vi "Autonomous Independent.vi"   [LabVIEW 2013]
doc: "This VI is called when autonomous begins, and will automatically be terminated when autonomous ends. You can carry out timed or sensor driven robot movement independently without needing to return to the caller."
uses:
  <vilib>/Rock Robotics/WPI/Solenoid/WPI_SolenoidValue.ctl
  Robot Global Data.vi
  <vilib>/Rock Robotics/WPI/RobotDrive/WPI_RobotDriveGetSetRefNum.vi
  <vilib>/Rock Robotics/WPI/Solenoid/WPI_SolenoidSetEnum.vi
  <vilib>/Rock Robotics/WPI/RobotDrive/WPI_RobotDriveArcadeDrive_Standard(NoSaturation).vi
  <vilib>/Rock Robotics/WPI/Solenoid/Deprecated/WPI_SolenoidGetBool.vi
  <vilib>/Rock Robotics/WPI/Joystick/WPI_JoystickGetSetRefNum.vi
panel:
  # "Be sure to right-click and choose Data Operations>>Make Current Value default if you want to save the array values with the VI"
types:
  T1 = typedef "WPI_JoystickDevRef.ctl" = cluster{"Device":T2}
  T2 = typedef "WPI_JoystickDeviceEnum.ctl" = enum16{"USB 1", "USB 2", "USB 3", "USB 4", "Kinect 1", "Kinect 2"}
  T3 = cluster{"axis 1 (x)":dbl, "axis 2 (y)":dbl, "axis 3 (throttle)":dbl, "axis 4":dbl, "axis 5":dbl, "axis 6":dbl}
  T4 = typedef "WPI_SolenoidValue.ctl" = enum16{"Off", "On", "Forward", "Reverse"}
  T5 = typedef "WPI_MotorControlDeviceRef.ctl" = cluster{"DeviceStatus":errorcluster, "Type":enum16{"PWM", "CAN"}, "PWM":cluster{"Digital Module":T6, "PWM Channel":T7, "DeadBand":T8}, "CAN":cluster{"Device Number":u8, "Control Mode":T9, "Semaphore":T10, "Max Vout":dbl}, "Invert":bool, "TransformRef":T11, "InvTransformRef":T11}
  T6 = typedef "FPGA_TypedefDigitalModule.ctl" = enum16{"Digital Module 1", "Digital Module 2"}
  T7 = typedef "FPGA_DIOPWMChannel.ctl" = enum8{"PWM 1", "PWM 2", "PWM 3", "PWM 4", "PWM 5", "PWM 6", "PWM 7", "PWM 8", "PWM 9", "PWM 10", "Invalid"}
  T8 = typedef "WPI_PWMDeadband.ctl" = cluster{"Name":string, "maxPositivePwm":i32, "minPositivePwm":i32, "centerPwm":i32, "maxNegativePwm":i32, "minNegativePwm":i32, "angularRange":u16}
  T9 = typedef "WPI_CANJaguar_ControlMode.ctl" = enum8{"Percent VBus", "Current", "Speed", "Position", "Voltage"}
  T10 = typedef "Semaphore RefNum" = refnum<k1>
  T11 = typedef "WPI_PWMTransform_ConPane.ctl" = refnum<vi>
  T12 = typedef "WPI_SolenoidDevRef.ctl" = cluster{"DevStatus":errorcluster, "Solenoid Module":T13, "Forward Solenoid Channel":T14, "Reverse Solenoid Channel":T14}
  T13 = typedef "FPGA_TypedefSolenoidModule.ctl" = enum16{"Solenoid Module 1", "Solenoid Module 2"}
  T14 = typedef "WPI_SolenoidChannel.ctl" = enum8{"Solenoid 1", "Solenoid 2", "Solenoid 3", "Solenoid 4", "Solenoid 5", "Solenoid 6", "Solenoid 7", "Solenoid 8", "Invalid"}
  T15 = typedef "WPI_DigitalInputDevRef.ctl" = cluster{"DevStatus":errorcluster, "DIO Channel":T16, "Digital Module":T6}
  T16 = typedef "FPGA_DIOChannel.ctl" = enum8{"DIO 1", "DIO 2", "DIO 3", "DIO 4", "DIO 5", "DIO 6", "DIO 7", "DIO 8", "DIO 9", "DIO 10", "DIO 11", "DIO 12", "DIO 13", "DIO 14", "Invalid"}
  T17 = typedef "WPI_RobotDriveDevRef.ctl" = cluster{"DevStatus":errorcluster, "Motors[]":T5[], "Square Inputs":bool, "Max Output":dbl, "Isochronous":bool}
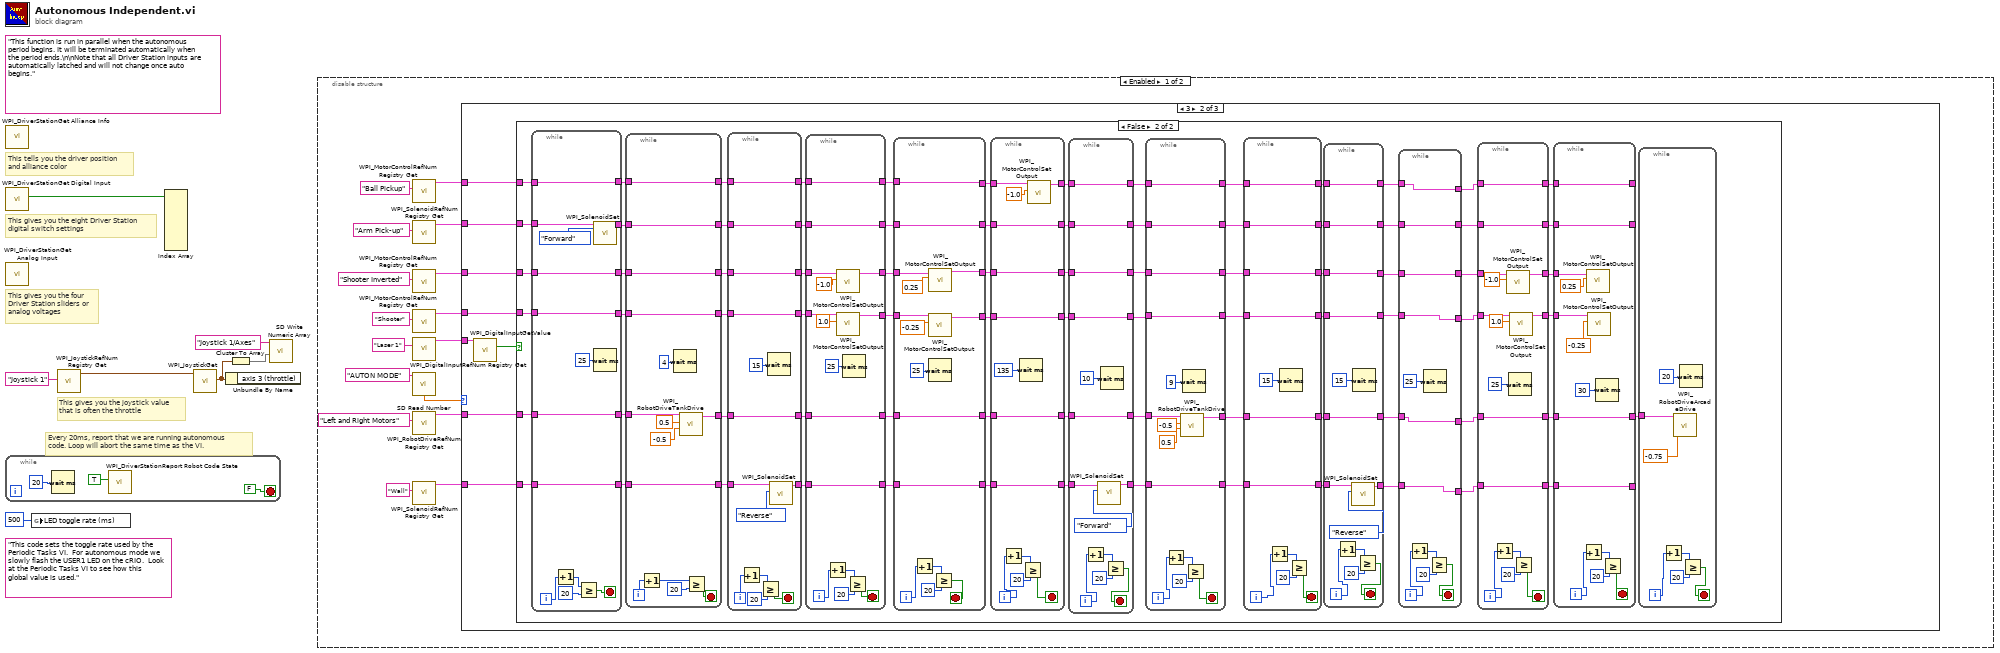
[diagram p0: block diagram]
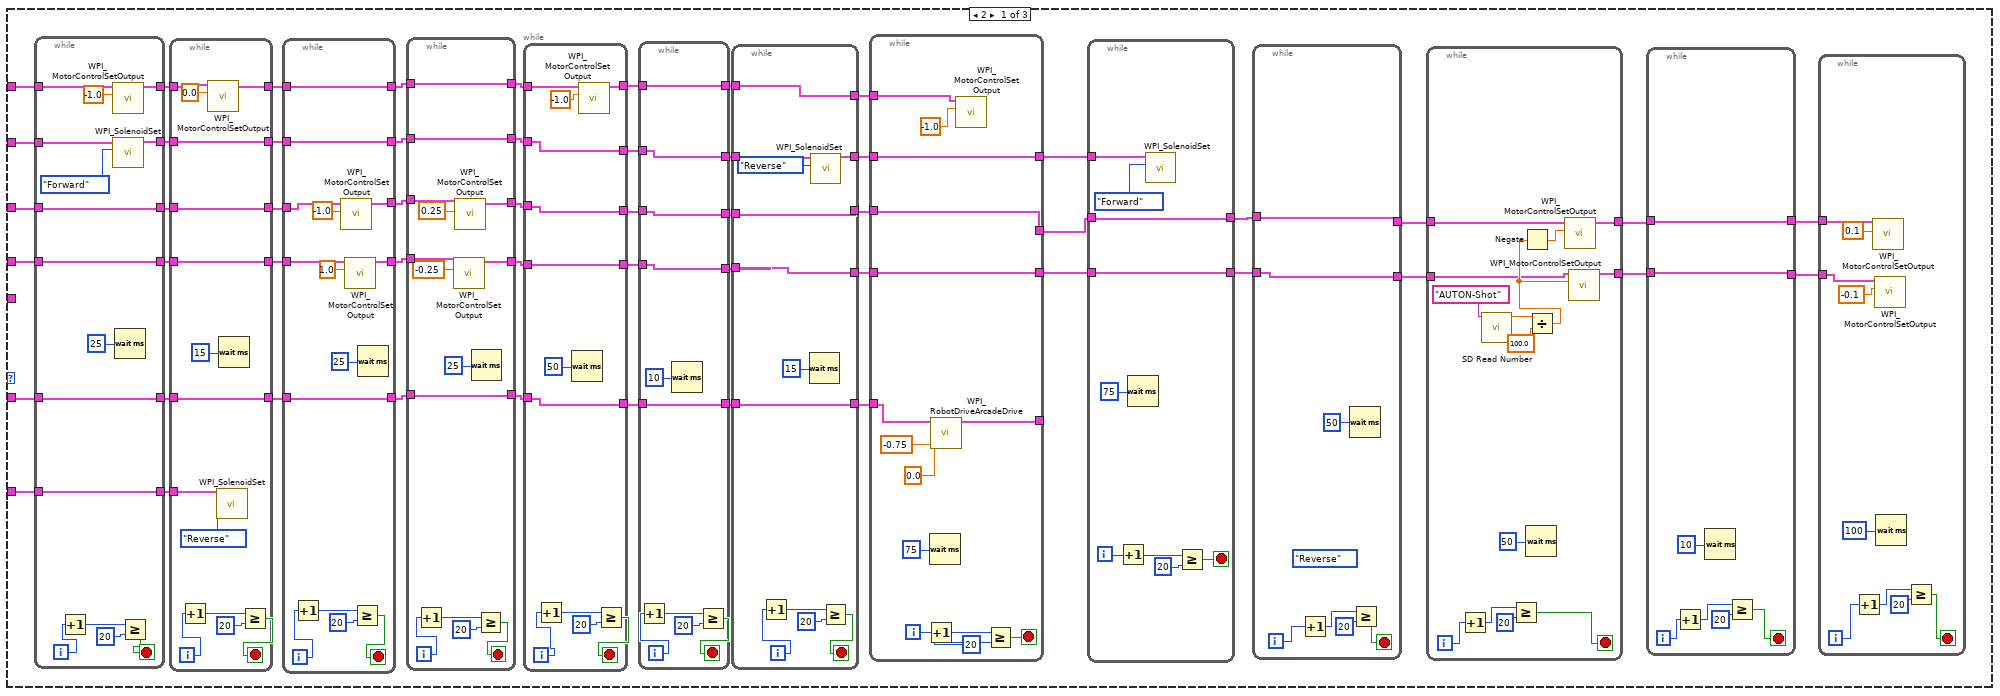
[diagram p2: hidden frame]
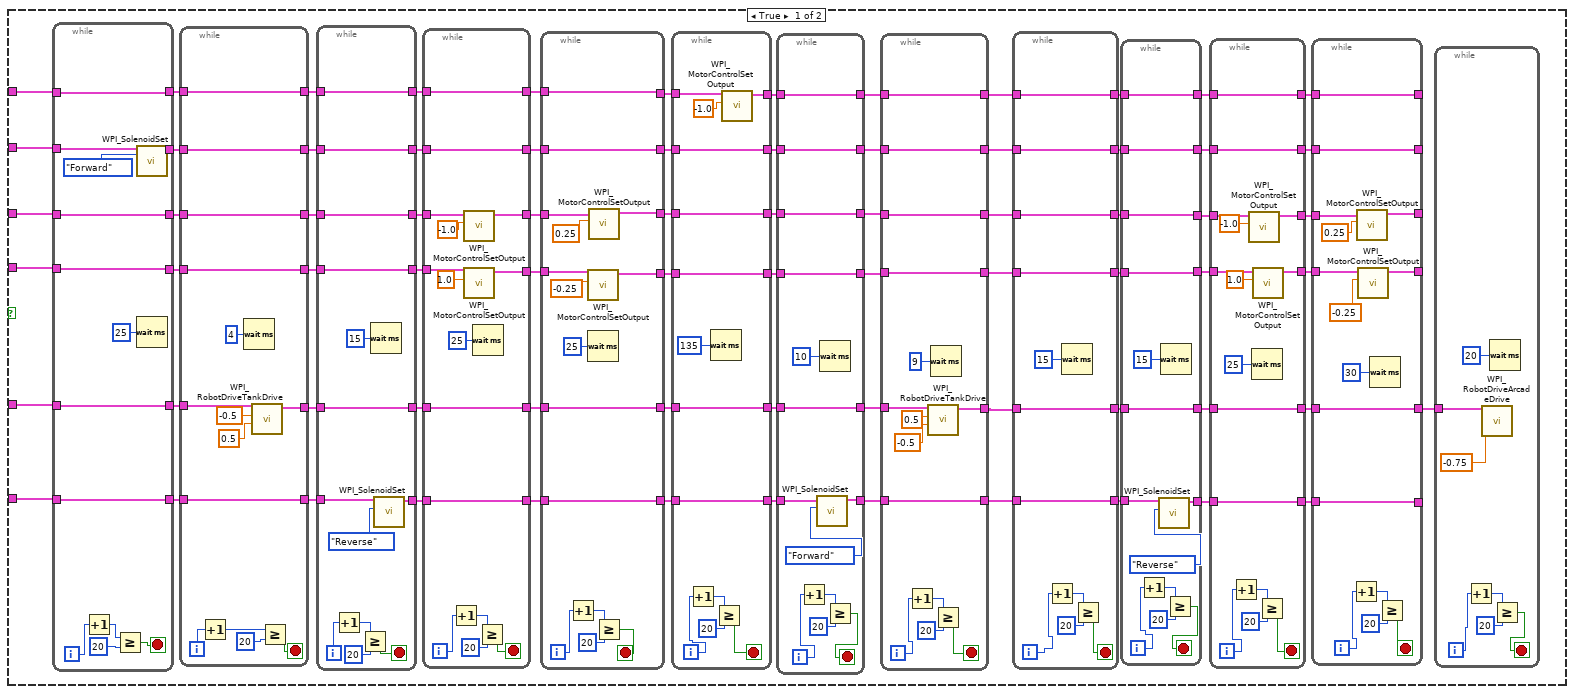
[diagram p3: hidden frame]
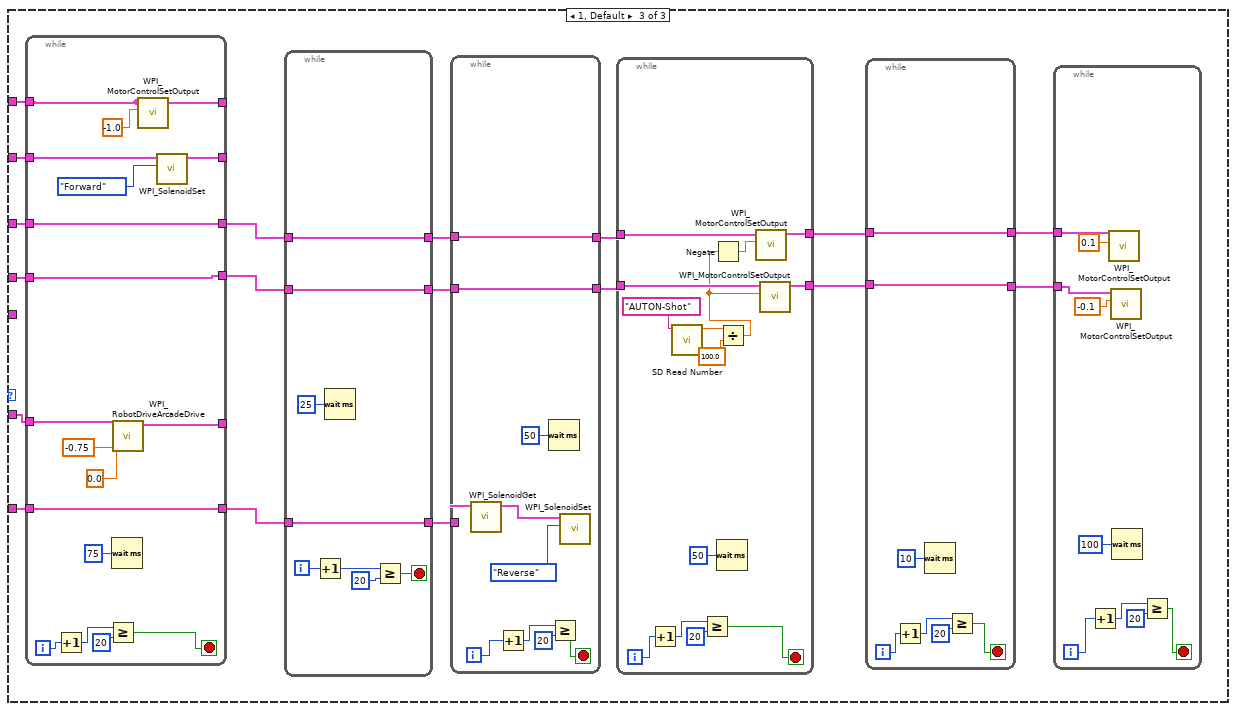
[diagram p4: hidden frame]
diagram:
  (unwired) "This code sets the toggle rate used by the Periodic Tasks VI.  For autonomous mode we slowly flash the USER1 LED on the cRIO.  Look at the Periodic Tasks VI to see how this global value is used."
  (unwired) "This function is run in parallel when the autonomous period begins. It will be terminated automatically when the period ends.\n\nNote that all Driver Station inputs are automatically latched and will not change once auto begins."
  # "Every 20ms, report that we are running autonomous\ncode. Loop will abort the same time as the VI."
  # "This gives you the joystick value\nthat is often the throttle"
  # "This tells you the driver position\nand alliance color"
  # "This gives you the eight Driver Station\ndigital switch settings"
  # "This gives you the four\nDriver Station sliders or\nanalog voltages"
  n1 = call <vilib>:"WPI_DriverStationGet Alliance Info.vi"() -> ()  [unwired: 12 out]
  n2 = call <vilib>:"WPI_DriverStationGet Digital Input.vi"() -> ("Driver Station Digital Input (1-8)"=w7:bool[])  [unwired: 11 out]
  n3 = call <vilib>:"WPI_DriverStationGet Analog Input.vi"() -> ()  [unwired: 12 out]
  n4 = while {
    stop <- FALSE stop-if-true
    n5 = Wait (ms)(milliseconds to wait=u32 20) -> ()  [unwired: 1 out]
    n6 = call <vilib>:"WPI_DriverStationReport Robot Code State.vi"("Autonomous"=TRUE) -> ()  [unwired: 10 in, 1 out]
  }
  n7 = global write "Robot Global Data.vi" "LED toggle rate (ms)"(u32 500 ("LED ms toggle rate")) -> ()
  n8 = call <vilib>:"WPI_JoystickRefNum Registry Get.vi"("refnum name"="Joystick 1") -> ("JoystickDevRef"=w5:T1)  [unwired: 1 in, 9 out]
  n9 = Index Array(array=w7) -> ()  [unwired: 8 in, 8 out]
  n10 = call <vilib>:"WPI_JoystickGet.vi"("JoystickDevRef"=w5) -> ("Axes"=w2:T3)  [unwired: 1 in, 5 out]
  n11 = Unbundle By Name(w2) -> ()  [unwired: 1 out]
  n12 = Cluster To Array(cluster=w2) -> (array=w3:dbl[])
  n13 = call <vilib>:"SD Write Numeric Array.vi"("Numeric Array"=w3, "Name"="Joystick 1/Axes") -> ()  [unwired: 8 in, 2 out]
  n14 = disable-structure shown="Enabled" {
    frame Enabled {
      n15 = call <vilib>:"SD Read Number.vi"("Name"="AUTON MODE") -> ("Numeric"=w25:dbl)  [unwired: 8 in, 2 out]
      n16 = call <vilib>:"WPI_MotorControlRefNum Registry Get.vi"("refnum name"="Ball Pickup") -> ("MotorControlDevRef"=w13:T5)  [unwired: 9 in, 1 out]
      n17 = call <vilib>:"WPI_SolenoidRefNum Registry Get.vi"("refnum name"="Arm Pick-up") -> ("SolenoidDevRef"=w14:T12)  [unwired: 9 in, 1 out]
      n18 = call <vilib>:"WPI_MotorControlRefNum Registry Get.vi"("refnum name"="Shooter Inverted") -> ("MotorControlDevRef"=w15:T5)  [unwired: 9 in, 1 out]
      n19 = call <vilib>:"WPI_MotorControlRefNum Registry Get.vi"("refnum name"="Shooter") -> ("MotorControlDevRef"=w16:T5)  [unwired: 9 in, 1 out]
      n20 = call <vilib>:"WPI_DigitalInputRefNum Registry Get.vi"("refnum name"="Laser 1") -> ("DigitalInputDevRef"=w12:T15)  [unwired: 9 in, 1 out]
      n21 = call <vilib>:"WPI_RobotDriveRefNum Registry Get.vi"("refnum name"="Left and Right Motors") -> ("RobotDriveDevRef"=w18:T17)  [unwired: 9 in, 1 out]
      n22 = call <vilib>:"WPI_SolenoidRefNum Registry Get.vi"("refnum name"="Wall") -> ("SolenoidDevRef"=w17:T12)  [unwired: 9 in, 1 out]
      n23 = case shown="3" w25 {
        tunnel: w18 -> [w71 w232 w759]
        tunnel: w17 -> [w70 w231 w748]
        tunnel: w16 -> [w72 w233 w758]
        tunnel: w15 -> [w73 w234 w757]
        tunnel: w14 -> [w75 w236 w756]
        tunnel: w13 -> [w74 w235 w755]
        tunnel: w12 -> [_ w238 _]
        frame 2 {
          n24 = while {
            tunnel: w75 -> [w166]
            tunnel: w74 -> [w164]
            tunnel: [w162] -> w66
            tunnel: w73 -> [w162]
            tunnel: w72 -> [w161]
            tunnel: [w161] -> w67
            tunnel: w71 -> [w160]
            tunnel: [w160] -> w68
            tunnel: w70 -> [w159]
            tunnel: [w159] -> w69
            tunnel: [w157] -> w65
            tunnel: [w156] -> w64
            i -> [w167]
            stop <- w168 stop-if-true
            n25 = Increment(x=w167) -> (x+1=w170:i32)
            n26 = call <vilib>:"WPI_MotorControlSetOutput.vi"("Output"=-1.0, "MotorControlDevRef"=w164) -> ("MotorControlDevRef"=w156:T5)  [unwired: 7 in, 2 out]
            n27 = call-poly <vilib>:"WPI_SolenoidSet.vi"("Value"=WPI_SolenoidValue."Forward", "SolenoidDevRef"=w166) -> ("SolenoidDevRef"=w157:T12)  [unwired: 8 in, 1 out]
            n28 = Wait (ms)(milliseconds to wait=u32 25) -> ()  [unwired: 1 out]
            n29 = Greater Or Equal?(x=w170, y=20) -> (x >= y?=w168:bool)
          }
          n30 = while {
            tunnel: w69 -> [w155]
            tunnel: w68 -> [w148]
            tunnel: w67 -> [w147]
            tunnel: w66 -> [w146]
            tunnel: w65 -> [w145]
            tunnel: w64 -> [w144]
            tunnel: [w148] -> w59
            tunnel: [w147] -> w60
            tunnel: [w146] -> w61
            tunnel: [w145] -> w62
            tunnel: [w143] -> w63
            i -> [w150]
            stop <- w151 stop-if-true
            n31 = Increment(x=w150) -> (x+1=w152:i32)
            n32 = call <vilib>:"WPI_MotorControlSetOutput.vi"("Output"=0.0, "MotorControlDevRef"=w144) -> ("MotorControlDevRef"=w143:T5)  [unwired: 7 in, 2 out]
            n33 = call-poly <vilib>:"WPI_SolenoidSet.vi"("Value"=WPI_SolenoidValue."Reverse", "SolenoidDevRef"=w155) -> ()  [unwired: 8 in, 2 out]
            n34 = Wait (ms)(milliseconds to wait=u32 15) -> ()  [unwired: 1 out]
            n35 = Greater Or Equal?(x=w152, y=20) -> (x >= y?=w151:bool)
          }
          n36 = while {
            tunnel: w63 -> [w141]
            tunnel: w62 -> [w140]
            tunnel: w61 -> [w138]
            tunnel: w60 -> [w139]
            tunnel: w59 -> [w135]
            tunnel: [w141] -> w58
            tunnel: [w140] -> w57
            tunnel: [w135] -> w54
            tunnel: [w134] -> w56
            tunnel: [w133] -> w55
            i -> [w129]
            stop <- w130 stop-if-true
            n37 = Increment(x=w129) -> (x+1=w132:i32)
            n38 = call <vilib>:"WPI_MotorControlSetOutput.vi"("Output"=-1.0, "MotorControlDevRef"=w138) -> ("MotorControlDevRef"=w134:T5)  [unwired: 7 in, 2 out]
            n39 = call <vilib>:"WPI_MotorControlSetOutput.vi"("Output"=1.0, "MotorControlDevRef"=w139) -> ("MotorControlDevRef"=w133:T5)  [unwired: 7 in, 2 out]
            n40 = Greater Or Equal?(x=w132, y=20) -> (x >= y?=w130:bool)
            n41 = Wait (ms)(milliseconds to wait=u32 25) -> ()  [unwired: 1 out]
          }
          n42 = while {
            tunnel: w58 -> [w123]
            tunnel: w57 -> [w122]
            tunnel: w56 -> [w126]
            tunnel: w55 -> [w127]
            tunnel: [w123] -> w49
            tunnel: [w122] -> w50
            tunnel: w54 -> [w121]
            tunnel: [w121] -> w53
            tunnel: [w120] -> w52
            tunnel: [w119] -> w51
            i -> [w115]
            stop <- w116 stop-if-true
            n43 = Increment(x=w115) -> (x+1=w117:i32)
            n44 = call <vilib>:"WPI_MotorControlSetOutput.vi"("Output"=-0.25, "MotorControlDevRef"=w127) -> ("MotorControlDevRef"=w120:T5)  [unwired: 7 in, 2 out]
            n45 = call <vilib>:"WPI_MotorControlSetOutput.vi"("Output"=0.25, "MotorControlDevRef"=w126) -> ("MotorControlDevRef"=w119:T5)  [unwired: 7 in, 2 out]
            n46 = Wait (ms)(milliseconds to wait=u32 25) -> ()  [unwired: 1 out]
            n47 = Greater Or Equal?(x=w117, y=20) -> (x >= y?=w116:bool)
          }
          n48 = while {
            tunnel: w53 -> [w106]
            tunnel: w52 -> [w105]
            tunnel: w51 -> [w104]
            tunnel: w50 -> [w103]
            tunnel: w49 -> [w113]
            tunnel: [w106] -> w44
            tunnel: [w105] -> w45
            tunnel: [w104] -> w46
            tunnel: [w103] -> w48
            tunnel: [w102] -> w47
            i -> [w108]
            stop <- w109 stop-if-true
            n49 = Increment(x=w108) -> (x+1=w111:i32)
            n50 = Wait (ms)(milliseconds to wait=u32 50) -> ()  [unwired: 1 out]
            n51 = call <vilib>:"WPI_MotorControlSetOutput.vi"("Output"=-1.0, "MotorControlDevRef"=w113) -> ("MotorControlDevRef"=w102:T5)  [unwired: 7 in, 2 out]
            n52 = Greater Or Equal?(x=w111, y=20) -> (x >= y?=w109:bool)
          }
          n53 = while {
            tunnel: w48 -> [w93]
            tunnel: w47 -> [w92]
            tunnel: w46 -> [w94]
            tunnel: w45 -> [w95]
            tunnel: w44 -> [w96]
            tunnel: [w96] -> w43
            tunnel: [w95] -> w41
            tunnel: [w94] -> w40
            tunnel: [w93] -> w39
            tunnel: [w92] -> w36
            i -> [w98]
            stop <- w97 stop-if-true
            n54 = Increment(x=w98) -> (x+1=w99:i32)
            n55 = Wait (ms)(milliseconds to wait=u32 10) -> ()  [unwired: 1 out]
            n56 = Greater Or Equal?(x=w99, y=20) -> (x >= y?=w97:bool)
          }
          n57 = while {
            tunnel: [w91] -> w42
            tunnel: w43 -> [w91]
            tunnel: w41 -> [w90]
            tunnel: [w90] -> w32
            tunnel: [w89] -> w31
            tunnel: w40 -> [w89]
            tunnel: w39 -> [w83]
            tunnel: [w82] -> w38
            tunnel: [w88] -> w37
            tunnel: w36 -> [w88]
            i -> [w84]
            stop <- w85 stop-if-true
            n58 = Increment(x=w84) -> (x+1=w87:i32)
            n59 = Wait (ms)(milliseconds to wait=u32 15) -> ()  [unwired: 1 out]
            n60 = call-poly <vilib>:"WPI_SolenoidSet.vi"("Value"=WPI_SolenoidValue."Reverse", "SolenoidDevRef"=w83) -> ("SolenoidDevRef"=w82:T12)  [unwired: 8 in, 1 out]
            n61 = Greater Or Equal?(x=w87, y=20) -> (x >= y?=w85:bool)
          }
          n62 = while {
            tunnel: [w225] -> _
            tunnel: w42 -> [w221]
            tunnel: w38 -> [w217]
            tunnel: w37 -> [w220]
            tunnel: [w219] -> w33
            tunnel: w32 -> [w219]
            tunnel: w31 -> [w218]
            tunnel: [w218] -> w30
            tunnel: [w217] -> w27
            i -> [w230]
            stop <- w227 stop-if-true
            n63 = Increment(x=w230) -> (x+1=w229:i32)
            n64 = Wait (ms)(milliseconds to wait=u32 75) -> ()  [unwired: 1 out]
            n65 = call-poly <vilib>:"WPI_RobotDriveArcadeDrive.vi"("Y axis value"=-0.75, "X axis value"=0.0, "RobotDriveDevRef"=w221) -> ("RobotDriveDevRef"=w225:T17)  [unwired: 6 in, 2 out]
            n66 = call <vilib>:"WPI_MotorControlSetOutput.vi"("Output"=-1.0, "MotorControlDevRef"=w220) -> ()  [unwired: 7 in, 3 out]
            n67 = Greater Or Equal?(x=w229, y=20) -> (x >= y?=w227:bool)
          }
          n68 = while {
            tunnel: [w174] -> w34
            tunnel: w33 -> [w174]
            tunnel: w30 -> [w173]
            tunnel: [w173] -> w29
            tunnel: w27 -> [w172]
            i -> [w177]
            stop <- w176 stop-if-true
            n69 = Increment(x=w177) -> (x+1=w178:i32)
            n70 = Wait (ms)(milliseconds to wait=u32 75) -> ()  [unwired: 1 out]
            n71 = call-poly <vilib>:"WPI_SolenoidSet.vi"("Value"=WPI_SolenoidValue."Forward", "SolenoidDevRef"=w172) -> ()  [unwired: 8 in, 2 out]
            n72 = Greater Or Equal?(x=w178, y=20) -> (x >= y?=w176:bool)
          }
          n73 = while {
            tunnel: [w211] -> w35
            tunnel: w34 -> [w211]
            tunnel: w29 -> [w210]
            tunnel: [w210] -> w28
            i -> [w214]
            stop <- w213 stop-if-true
            (unwired) WPI_SolenoidValue."Reverse" ("Value")
            n74 = Increment(x=w214) -> (x+1=w215:i32)
            n75 = Wait (ms)(milliseconds to wait=u32 50) -> ()  [unwired: 1 out]
            n76 = Greater Or Equal?(x=w215, y=20) -> (x >= y?=w213:bool)
          }
          n77 = while {
            tunnel: [w205] -> w79
            tunnel: [w204] -> w78
            tunnel: w35 -> [w197]
            tunnel: w28 -> [w196]
            i -> [w207]
            stop <- w206 stop-if-true
            n78 = Increment(x=w207) -> (x+1=w209:i32)
            n79 = call <vilib>:"SD Read Number.vi"("Name"="AUTON-Shot") -> ("Numeric"=w200:dbl)  [unwired: 8 in, 2 out]
            n80 = Greater Or Equal?(x=w209, y=20) -> (x >= y?=w206:bool)
            n81 = Wait (ms)(milliseconds to wait=u32 50) -> ()  [unwired: 1 out]
            n82 = Divide(x=w200, y=100.0) -> (x/y=w199:dbl)
            n83 = Negate(x=w199) -> (-x=w201:dbl)
            n84 = call <vilib>:"WPI_MotorControlSetOutput.vi"("Output"=w201, "MotorControlDevRef"=w196) -> ("MotorControlDevRef"=w204:T5)  [unwired: 7 in, 2 out]
            n85 = call <vilib>:"WPI_MotorControlSetOutput.vi"("Output"=w199, "MotorControlDevRef"=w197) -> ("MotorControlDevRef"=w205:T5)  [unwired: 7 in, 2 out]
          }
          n86 = while {
            tunnel: w79 -> [w191]
            tunnel: w78 -> [w190]
            tunnel: [w191] -> w76
            tunnel: [w190] -> w77
            i -> [w192]
            stop <- w193 stop-if-true
            n87 = Increment(x=w192) -> (x+1=w194:i32)
            n88 = Wait (ms)(milliseconds to wait=u32 10) -> ()  [unwired: 1 out]
            n89 = Greater Or Equal?(x=w194, y=20) -> (x >= y?=w193:bool)
          }
          n90 = while {
            tunnel: w77 -> [w187]
            tunnel: w76 -> [w188]
            i -> [w182]
            stop <- w181 stop-if-true
            n91 = Increment(x=w182) -> (x+1=w184:i32)
            n92 = call <vilib>:"WPI_MotorControlSetOutput.vi"("Output"=0.1, "MotorControlDevRef"=w187) -> ()  [unwired: 7 in, 3 out]
            n93 = call <vilib>:"WPI_MotorControlSetOutput.vi"("Output"=-0.1, "MotorControlDevRef"=w188) -> ()  [unwired: 7 in, 3 out]
            n94 = Wait (ms)(milliseconds to wait=u32 100) -> ()  [unwired: 1 out]
            n95 = Greater Or Equal?(x=w184, y=20) -> (x >= y?=w181:bool)
          }
        }
        frame 3 {
          n96 = call <vilib>:"WPI_DigitalInputGetValue.vi"("DigitalInputDevRef"=w238) -> ("Value"=w237:bool)  [unwired: 8 in, 2 out]
          n97 = case shown="False" w237 {
            tunnel: w236 -> [w244 w561]
            tunnel: w235 -> [w245 w556]
            tunnel: w234 -> [w243 w557]
            tunnel: w233 -> [w242 w558]
            tunnel: w232 -> [w241 w559]
            tunnel: w231 -> [w240 w560]
            frame True {
              n98 = while {
                tunnel: w244 -> [w478]
                tunnel: [w476] -> w309
                tunnel: w240 -> [w474]
                tunnel: [w474] -> w306
                tunnel: w241 -> [w473]
                tunnel: [w473] -> w307
                tunnel: [w472] -> w311
                tunnel: w242 -> [w472]
                tunnel: w243 -> [w471]
                tunnel: [w471] -> w310
                tunnel: [w470] -> w308
                tunnel: w245 -> [w470]
                i -> [w480]
                stop <- w479 stop-if-true
                n99 = Increment(x=w480) -> (x+1=w482:i32)
                n100 = Greater Or Equal?(x=w482, y=20) -> (x >= y?=w479:bool)
                n101 = call-poly <vilib>:"WPI_SolenoidSet.vi"("Value"=WPI_SolenoidValue."Forward", "SolenoidDevRef"=w478) -> ("SolenoidDevRef"=w476:T12)  [unwired: 8 in, 1 out]
                n102 = Wait (ms)(milliseconds to wait=u32 25) -> ()  [unwired: 1 out]
              }
              n103 = while {
                tunnel: w311 -> [w461]
                tunnel: w310 -> [w460]
                tunnel: w309 -> [w459]
                tunnel: w308 -> [w458]
                tunnel: w307 -> [w465]
                tunnel: w306 -> [w463]
                tunnel: [w463] -> w300
                tunnel: [w462] -> w301
                tunnel: [w461] -> w302
                tunnel: [w460] -> w303
                tunnel: [w459] -> w304
                tunnel: [w458] -> w305
                i -> [w466]
                stop <- w467 stop-if-true
                n104 = Increment(x=w466) -> (x+1=w468:i32)
                n105 = Wait (ms)(milliseconds to wait=u32 4) -> ()  [unwired: 1 out]
                n106 = call <vilib>:"WPI_RobotDriveTankDrive.vi"("Right axis value"=0.5, "Left axis value"=-0.5, "RobotDriveDevRef"=w465) -> ("RobotDriveDevRef"=w462:T17)  [unwired: 6 in, 2 out]
                n107 = Greater Or Equal?(x=w468, y=20) -> (x >= y?=w467:bool)
              }
              n108 = while {
                tunnel: w305 -> [w449]
                tunnel: w304 -> [w450]
                tunnel: w303 -> [w451]
                tunnel: w302 -> [w452]
                tunnel: w301 -> [w453]
                tunnel: w300 -> [w455]
                tunnel: [w453] -> w295
                tunnel: [w452] -> w296
                tunnel: [w451] -> w297
                tunnel: [w450] -> w298
                tunnel: [w449] -> w299
                tunnel: [w448] -> w294
                i -> [w447]
                stop <- w444 stop-if-true
                n109 = Increment(x=w447) -> (x+1=w446:i32)
                n110 = Greater Or Equal?(x=w446, y=20) -> (x >= y?=w444:bool)
                n111 = Wait (ms)(milliseconds to wait=u32 15) -> ()  [unwired: 1 out]
                n112 = call-poly <vilib>:"WPI_SolenoidSet.vi"("Value"=WPI_SolenoidValue."Reverse", "SolenoidDevRef"=w455) -> ("SolenoidDevRef"=w448:T12)  [unwired: 8 in, 1 out]
              }
              n113 = while {
                tunnel: w299 -> [w429]
                tunnel: w298 -> [w430]
                tunnel: w297 -> [w441]
                tunnel: w296 -> [w442]
                tunnel: w295 -> [w434]
                tunnel: w294 -> [w433]
                tunnel: [w434] -> w292
                tunnel: [w433] -> w293
                tunnel: [w432] -> w290
                tunnel: [w431] -> w291
                tunnel: [w430] -> w289
                tunnel: [w429] -> w288
                i -> [w435]
                stop <- w436 stop-if-true
                n114 = Increment(x=w435) -> (x+1=w437:i32)
                n115 = call <vilib>:"WPI_MotorControlSetOutput.vi"("Output"=-1.0, "MotorControlDevRef"=w441) -> ("MotorControlDevRef"=w432:T5)  [unwired: 7 in, 2 out]
                n116 = call <vilib>:"WPI_MotorControlSetOutput.vi"("Output"=1.0, "MotorControlDevRef"=w442) -> ("MotorControlDevRef"=w431:T5)  [unwired: 7 in, 2 out]
                n117 = Wait (ms)(milliseconds to wait=u32 25) -> ()  [unwired: 1 out]
                n118 = Greater Or Equal?(x=w437, y=20) -> (x >= y?=w436:bool)
              }
              n119 = while {
                tunnel: w293 -> [w413]
                tunnel: w292 -> [w414]
                tunnel: w291 -> [w426]
                tunnel: w290 -> [w427]
                tunnel: w289 -> [w417]
                tunnel: w288 -> [w418]
                tunnel: [w418] -> w282
                tunnel: [w417] -> w283
                tunnel: [w416] -> w284
                tunnel: [w415] -> w285
                tunnel: [w414] -> w286
                tunnel: [w413] -> w287
                i -> [w419]
                stop <- w420 stop-if-true
                n120 = Increment(x=w419) -> (x+1=w422:i32)
                n121 = call <vilib>:"WPI_MotorControlSetOutput.vi"("Output"=-0.25, "MotorControlDevRef"=w426) -> ("MotorControlDevRef"=w415:T5)  [unwired: 7 in, 2 out]
                n122 = Wait (ms)(milliseconds to wait=u32 25) -> ()  [unwired: 1 out]
                n123 = call <vilib>:"WPI_MotorControlSetOutput.vi"("Output"=0.25, "MotorControlDevRef"=w427) -> ("MotorControlDevRef"=w416:T5)  [unwired: 7 in, 2 out]
                n124 = Greater Or Equal?(x=w422, y=20) -> (x >= y?=w420:bool)
              }
              n125 = while {
                tunnel: w287 -> [w404]
                tunnel: w286 -> [w409]
                tunnel: w285 -> [w408]
                tunnel: w284 -> [w407]
                tunnel: w283 -> [w406]
                tunnel: w282 -> [w412]
                tunnel: [w409] -> w277
                tunnel: [w408] -> w278
                tunnel: [w407] -> w279
                tunnel: [w406] -> w281
                tunnel: [w405] -> w280
                tunnel: [w404] -> w276
                i -> [w400]
                stop <- w401 stop-if-true
                n126 = Increment(x=w400) -> (x+1=w402:i32)
                n127 = Wait (ms)(milliseconds to wait=u32 135) -> ()  [unwired: 1 out]
                n128 = Greater Or Equal?(x=w402, y=20) -> (x >= y?=w401:bool)
                n129 = call <vilib>:"WPI_MotorControlSetOutput.vi"("Output"=-1.0, "MotorControlDevRef"=w412) -> ("MotorControlDevRef"=w405:T5)  [unwired: 7 in, 2 out]
              }
              n130 = while {
                tunnel: w281 -> [w397]
                tunnel: w280 -> [w396]
                tunnel: w279 -> [w398]
                tunnel: w278 -> [w394]
                tunnel: w277 -> [w395]
                tunnel: w276 -> [w388]
                tunnel: [w398] -> w255
                tunnel: [w397] -> w256
                tunnel: [w396] -> w257
                tunnel: [w395] -> w253
                tunnel: [w387] -> w252
                tunnel: [w394] -> w254
                i -> [w390]
                stop <- w391 stop-if-true
                n131 = Increment(x=w390) -> (x+1=w393:i32)
                n132 = call-poly <vilib>:"WPI_SolenoidSet.vi"("Value"=WPI_SolenoidValue."Forward", "SolenoidDevRef"=w388) -> ("SolenoidDevRef"=w387:T12)  [unwired: 8 in, 1 out]
                n133 = Wait (ms)(milliseconds to wait=u32 10) -> ()  [unwired: 1 out]
                n134 = Greater Or Equal?(x=w393, y=20) -> (x >= y?=w391:bool)
              }
              n135 = while {
                tunnel: w257 -> [w374]
                tunnel: w256 -> [w375]
                tunnel: w255 -> [w376]
                tunnel: w254 -> [w377]
                tunnel: w253 -> [w386]
                tunnel: w252 -> [w378]
                tunnel: [w379] -> w247
                tunnel: [w378] -> w246
                tunnel: [w377] -> w251
                tunnel: [w376] -> w250
                tunnel: [w375] -> w249
                tunnel: [w374] -> w248
                i -> [w381]
                stop <- w382 stop-if-true
                n136 = Increment(x=w381) -> (x+1=w384:i32)
                n137 = call <vilib>:"WPI_RobotDriveTankDrive.vi"("Right axis value"=-0.5, "Left axis value"=0.5, "RobotDriveDevRef"=w386) -> ("RobotDriveDevRef"=w379:T17)  [unwired: 6 in, 2 out]
                n138 = Wait (ms)(milliseconds to wait=u32 9) -> ()  [unwired: 1 out]
                n139 = Greater Or Equal?(x=w384, y=20) -> (x >= y?=w382:bool)
              }
              n140 = while {
                tunnel: w248 -> [w368]
                tunnel: w249 -> [w362]
                tunnel: w250 -> [w367]
                tunnel: w251 -> [w366]
                tunnel: w247 -> [w365]
                tunnel: w246 -> [w364]
                tunnel: [w362] -> w271
                tunnel: [w368] -> w270
                tunnel: [w367] -> w272
                tunnel: [w366] -> w273
                tunnel: [w365] -> w274
                tunnel: [w364] -> w275
                i -> [w369]
                stop <- w370 stop-if-true
                n141 = Increment(x=w369) -> (x+1=w371:i32)
                n142 = Wait (ms)(milliseconds to wait=u32 15) -> ()  [unwired: 1 out]
                n143 = Greater Or Equal?(x=w371, y=20) -> (x >= y?=w370:bool)
              }
              n144 = while {
                tunnel: w275 -> [w361]
                tunnel: [w359] -> w268
                tunnel: w274 -> [w359]
                tunnel: [w358] -> w269
                tunnel: [w357] -> w267
                tunnel: w273 -> [w357]
                tunnel: [w356] -> w266
                tunnel: w272 -> [w356]
                tunnel: [w355] -> w265
                tunnel: w271 -> [w355]
                tunnel: [w354] -> w264
                tunnel: w270 -> [w354]
                i -> [w350]
                stop <- w351 stop-if-true
                n145 = Increment(x=w350) -> (x+1=w353:i32)
                n146 = call-poly <vilib>:"WPI_SolenoidSet.vi"("Value"=WPI_SolenoidValue."Reverse", "SolenoidDevRef"=w361) -> ("SolenoidDevRef"=w358:T12)  [unwired: 8 in, 1 out]
                n147 = Wait (ms)(milliseconds to wait=u32 15) -> ()  [unwired: 1 out]
                n148 = Greater Or Equal?(x=w353, y=20) -> (x >= y?=w351:bool)
              }
              n149 = while {
                tunnel: w269 -> [w340]
                tunnel: w268 -> [w339]
                tunnel: w267 -> [w344]
                tunnel: w266 -> [w343]
                tunnel: w265 -> [w336]
                tunnel: w264 -> [w335]
                tunnel: [w340] -> w261
                tunnel: [w339] -> w260
                tunnel: [w338] -> w263
                tunnel: [w337] -> w262
                tunnel: [w336] -> w259
                tunnel: [w335] -> w258
                i -> [w345]
                stop <- w346 stop-if-true
                n150 = Increment(x=w345) -> (x+1=w347:i32)
                n151 = call <vilib>:"WPI_MotorControlSetOutput.vi"("Output"=-1.0, "MotorControlDevRef"=w343) -> ("MotorControlDevRef"=w337:T5)  [unwired: 7 in, 2 out]
                n152 = Wait (ms)(milliseconds to wait=u32 25) -> ()  [unwired: 1 out]
                n153 = call <vilib>:"WPI_MotorControlSetOutput.vi"("Output"=1.0, "MotorControlDevRef"=w344) -> ("MotorControlDevRef"=w338:T5)  [unwired: 7 in, 2 out]
                n154 = Greater Or Equal?(x=w347, y=20) -> (x >= y?=w346:bool)
              }
              n155 = while {
                tunnel: w263 -> [w329]
                tunnel: w262 -> [w328]
                tunnel: [w325] -> _
                tunnel: w261 -> [w325]
                tunnel: w260 -> [w324]
                tunnel: [w324] -> w239
                tunnel: w259 -> [w323]
                tunnel: [w323] -> _
                tunnel: w258 -> [w322]
                tunnel: [w322] -> _
                tunnel: [w320] -> _
                tunnel: [w319] -> _
                i -> [w330]
                stop <- w331 stop-if-true
                n156 = Increment(x=w330) -> (x+1=w333:i32)
                n157 = call <vilib>:"WPI_MotorControlSetOutput.vi"("Output"=0.25, "MotorControlDevRef"=w328) -> ("MotorControlDevRef"=w319:T5)  [unwired: 7 in, 2 out]
                n158 = call <vilib>:"WPI_MotorControlSetOutput.vi"("Output"=-0.25, "MotorControlDevRef"=w329) -> ("MotorControlDevRef"=w320:T5)  [unwired: 7 in, 2 out]
                n159 = Wait (ms)(milliseconds to wait=u32 30) -> ()  [unwired: 1 out]
                n160 = Greater Or Equal?(x=w333, y=20) -> (x >= y?=w331:bool)
              }
              n161 = while {
                tunnel: w239 -> [w318]
                i -> [w313]
                stop <- w314 stop-if-true
                n162 = Increment(x=w313) -> (x+1=w315:i32)
                n163 = call-poly <vilib>:"WPI_RobotDriveArcadeDrive.vi"("Y axis value"=-0.75, "RobotDriveDevRef"=w318) -> ()  [unwired: 7 in, 3 out]
                n164 = Wait (ms)(milliseconds to wait=u32 20) -> ()  [unwired: 1 out]
                n165 = Greater Or Equal?(x=w315, y=20) -> (x >= y?=w314:bool)
              }
            }
            frame False {
              n166 = while {
                tunnel: w561 -> [w737]
                tunnel: [w735] -> w553
                tunnel: w560 -> [w733]
                tunnel: [w733] -> w550
                tunnel: w559 -> [w732]
                tunnel: [w732] -> w551
                tunnel: [w731] -> w555
                tunnel: w558 -> [w731]
                tunnel: w557 -> [w730]
                tunnel: [w730] -> w554
                tunnel: [w729] -> w552
                tunnel: w556 -> [w729]
                i -> [w739]
                stop <- w738 stop-if-true
                n167 = Increment(x=w739) -> (x+1=w741:i32)
                n168 = Greater Or Equal?(x=w741, y=20) -> (x >= y?=w738:bool)
                n169 = call-poly <vilib>:"WPI_SolenoidSet.vi"("Value"=WPI_SolenoidValue."Forward", "SolenoidDevRef"=w737) -> ("SolenoidDevRef"=w735:T12)  [unwired: 8 in, 1 out]
                n170 = Wait (ms)(milliseconds to wait=u32 25) -> ()  [unwired: 1 out]
              }
              n171 = while {
                tunnel: w555 -> [w720]
                tunnel: w554 -> [w719]
                tunnel: w553 -> [w718]
                tunnel: w552 -> [w717]
                tunnel: w551 -> [w724]
                tunnel: w550 -> [w722]
                tunnel: [w722] -> w544
                tunnel: [w721] -> w545
                tunnel: [w720] -> w546
                tunnel: [w719] -> w547
                tunnel: [w718] -> w548
                tunnel: [w717] -> w549
                i -> [w725]
                stop <- w726 stop-if-true
                n172 = Increment(x=w725) -> (x+1=w727:i32)
                n173 = Wait (ms)(milliseconds to wait=u32 4) -> ()  [unwired: 1 out]
                n174 = call <vilib>:"WPI_RobotDriveTankDrive.vi"("Right axis value"=-0.5, "Left axis value"=0.5, "RobotDriveDevRef"=w724) -> ("RobotDriveDevRef"=w721:T17)  [unwired: 6 in, 2 out]
                n175 = Greater Or Equal?(x=w727, y=20) -> (x >= y?=w726:bool)
              }
              n176 = while {
                tunnel: w549 -> [w708]
                tunnel: w548 -> [w709]
                tunnel: w547 -> [w710]
                tunnel: w546 -> [w711]
                tunnel: w545 -> [w712]
                tunnel: w544 -> [w714]
                tunnel: [w712] -> w539
                tunnel: [w711] -> w540
                tunnel: [w710] -> w541
                tunnel: [w709] -> w542
                tunnel: [w708] -> w543
                tunnel: [w707] -> w538
                i -> [w706]
                stop <- w703 stop-if-true
                n177 = Increment(x=w706) -> (x+1=w705:i32)
                n178 = Greater Or Equal?(x=w705, y=20) -> (x >= y?=w703:bool)
                n179 = Wait (ms)(milliseconds to wait=u32 15) -> ()  [unwired: 1 out]
                n180 = call-poly <vilib>:"WPI_SolenoidSet.vi"("Value"=WPI_SolenoidValue."Reverse", "SolenoidDevRef"=w714) -> ("SolenoidDevRef"=w707:T12)  [unwired: 8 in, 1 out]
              }
              n181 = while {
                tunnel: w543 -> [w688]
                tunnel: w542 -> [w689]
                tunnel: w541 -> [w700]
                tunnel: w540 -> [w701]
                tunnel: w539 -> [w693]
                tunnel: w538 -> [w692]
                tunnel: [w693] -> w536
                tunnel: [w692] -> w537
                tunnel: [w691] -> w534
                tunnel: [w690] -> w535
                tunnel: [w689] -> w533
                tunnel: [w688] -> w532
                i -> [w694]
                stop <- w695 stop-if-true
                n182 = Increment(x=w694) -> (x+1=w696:i32)
                n183 = call <vilib>:"WPI_MotorControlSetOutput.vi"("Output"=-1.0, "MotorControlDevRef"=w700) -> ("MotorControlDevRef"=w691:T5)  [unwired: 7 in, 2 out]
                n184 = call <vilib>:"WPI_MotorControlSetOutput.vi"("Output"=1.0, "MotorControlDevRef"=w701) -> ("MotorControlDevRef"=w690:T5)  [unwired: 7 in, 2 out]
                n185 = Wait (ms)(milliseconds to wait=u32 25) -> ()  [unwired: 1 out]
                n186 = Greater Or Equal?(x=w696, y=20) -> (x >= y?=w695:bool)
              }
              n187 = while {
                tunnel: w537 -> [w672]
                tunnel: w536 -> [w673]
                tunnel: w535 -> [w685]
                tunnel: w534 -> [w686]
                tunnel: w533 -> [w676]
                tunnel: w532 -> [w677]
                tunnel: [w677] -> w526
                tunnel: [w676] -> w527
                tunnel: [w675] -> w528
                tunnel: [w674] -> w529
                tunnel: [w673] -> w530
                tunnel: [w672] -> w531
                i -> [w678]
                stop <- w679 stop-if-true
                n188 = Increment(x=w678) -> (x+1=w681:i32)
                n189 = call <vilib>:"WPI_MotorControlSetOutput.vi"("Output"=-0.25, "MotorControlDevRef"=w685) -> ("MotorControlDevRef"=w674:T5)  [unwired: 7 in, 2 out]
                n190 = Wait (ms)(milliseconds to wait=u32 25) -> ()  [unwired: 1 out]
                n191 = call <vilib>:"WPI_MotorControlSetOutput.vi"("Output"=0.25, "MotorControlDevRef"=w686) -> ("MotorControlDevRef"=w675:T5)  [unwired: 7 in, 2 out]
                n192 = Greater Or Equal?(x=w681, y=20) -> (x >= y?=w679:bool)
              }
              n193 = while {
                tunnel: w531 -> [w663]
                tunnel: w530 -> [w668]
                tunnel: w529 -> [w667]
                tunnel: w528 -> [w666]
                tunnel: w527 -> [w665]
                tunnel: w526 -> [w671]
                tunnel: [w668] -> w521
                tunnel: [w667] -> w522
                tunnel: [w666] -> w523
                tunnel: [w665] -> w525
                tunnel: [w664] -> w524
                tunnel: [w663] -> w520
                i -> [w659]
                stop <- w660 stop-if-true
                n194 = Increment(x=w659) -> (x+1=w661:i32)
                n195 = Wait (ms)(milliseconds to wait=u32 135) -> ()  [unwired: 1 out]
                n196 = Greater Or Equal?(x=w661, y=20) -> (x >= y?=w660:bool)
                n197 = call <vilib>:"WPI_MotorControlSetOutput.vi"("Output"=-1.0, "MotorControlDevRef"=w671) -> ("MotorControlDevRef"=w664:T5)  [unwired: 7 in, 2 out]
              }
              n198 = while {
                tunnel: w525 -> [w656]
                tunnel: w524 -> [w655]
                tunnel: w523 -> [w657]
                tunnel: w522 -> [w653]
                tunnel: w521 -> [w654]
                tunnel: w520 -> [w647]
                tunnel: [w657] -> w505
                tunnel: [w656] -> w506
                tunnel: [w655] -> w507
                tunnel: [w654] -> w503
                tunnel: [w646] -> w502
                tunnel: [w653] -> w504
                i -> [w649]
                stop <- w650 stop-if-true
                n199 = Increment(x=w649) -> (x+1=w652:i32)
                n200 = call-poly <vilib>:"WPI_SolenoidSet.vi"("Value"=WPI_SolenoidValue."Forward", "SolenoidDevRef"=w647) -> ("SolenoidDevRef"=w646:T12)  [unwired: 8 in, 1 out]
                n201 = Wait (ms)(milliseconds to wait=u32 10) -> ()  [unwired: 1 out]
                n202 = Greater Or Equal?(x=w652, y=20) -> (x >= y?=w650:bool)
              }
              n203 = while {
                tunnel: w507 -> [w633]
                tunnel: w506 -> [w634]
                tunnel: w505 -> [w635]
                tunnel: w504 -> [w636]
                tunnel: w503 -> [w645]
                tunnel: w502 -> [w637]
                tunnel: [w638] -> w497
                tunnel: [w637] -> w496
                tunnel: [w636] -> w501
                tunnel: [w635] -> w500
                tunnel: [w634] -> w499
                tunnel: [w633] -> w498
                i -> [w640]
                stop <- w641 stop-if-true
                n204 = Increment(x=w640) -> (x+1=w643:i32)
                n205 = call <vilib>:"WPI_RobotDriveTankDrive.vi"("Right axis value"=0.5, "Left axis value"=-0.5, "RobotDriveDevRef"=w645) -> ("RobotDriveDevRef"=w638:T17)  [unwired: 6 in, 2 out]
                n206 = Wait (ms)(milliseconds to wait=u32 9) -> ()  [unwired: 1 out]
                n207 = Greater Or Equal?(x=w643, y=20) -> (x >= y?=w641:bool)
              }
              n208 = while {
                tunnel: w498 -> [w627]
                tunnel: w499 -> [w621]
                tunnel: w500 -> [w626]
                tunnel: w501 -> [w625]
                tunnel: w497 -> [w624]
                tunnel: w496 -> [w623]
                tunnel: [w621] -> w515
                tunnel: [w627] -> w514
                tunnel: [w626] -> w516
                tunnel: [w625] -> w517
                tunnel: [w624] -> w518
                tunnel: [w623] -> w519
                i -> [w628]
                stop <- w629 stop-if-true
                n209 = Increment(x=w628) -> (x+1=w630:i32)
                n210 = Wait (ms)(milliseconds to wait=u32 15) -> ()  [unwired: 1 out]
                n211 = Greater Or Equal?(x=w630, y=20) -> (x >= y?=w629:bool)
              }
              n212 = while {
                tunnel: w519 -> [w620]
                tunnel: [w618] -> w491
                tunnel: w518 -> [w618]
                tunnel: [w617] -> w493
                tunnel: [w616] -> w489
                tunnel: w517 -> [w616]
                tunnel: [w615] -> w487
                tunnel: w516 -> [w615]
                tunnel: [w614] -> w485
                tunnel: w515 -> [w614]
                tunnel: [w613] -> w483
                tunnel: w514 -> [w613]
                i -> [w609]
                stop <- w610 stop-if-true
                n213 = Increment(x=w609) -> (x+1=w612:i32)
                n214 = call-poly <vilib>:"WPI_SolenoidSet.vi"("Value"=WPI_SolenoidValue."Reverse", "SolenoidDevRef"=w620) -> ("SolenoidDevRef"=w617:T12)  [unwired: 8 in, 1 out]
                n215 = Wait (ms)(milliseconds to wait=u32 15) -> ()  [unwired: 1 out]
                n216 = Greater Or Equal?(x=w612, y=20) -> (x >= y?=w610:bool)
              }
              n217 = while {
                tunnel: [w568] -> w494
                tunnel: w493 -> [w568]
                tunnel: [w567] -> w492
                tunnel: w491 -> [w567]
                tunnel: [w566] -> w490
                tunnel: w489 -> [w566]
                tunnel: [w565] -> w488
                tunnel: w487 -> [w565]
                tunnel: [w564] -> w486
                tunnel: w485 -> [w564]
                tunnel: [w563] -> w484
                tunnel: w483 -> [w563]
                i -> [w569]
                stop <- w570 stop-if-true
                n218 = Increment(x=w569) -> (x+1=w572:i32)
                n219 = Wait (ms)(milliseconds to wait=u32 25) -> ()  [unwired: 1 out]
                n220 = Greater Or Equal?(x=w572, y=20) -> (x >= y?=w570:bool)
              }
              n221 = while {
                tunnel: w494 -> [w599]
                tunnel: w492 -> [w598]
                tunnel: w490 -> [w603]
                tunnel: w488 -> [w602]
                tunnel: w486 -> [w595]
                tunnel: w484 -> [w594]
                tunnel: [w599] -> w511
                tunnel: [w598] -> w510
                tunnel: [w597] -> w513
                tunnel: [w596] -> w512
                tunnel: [w595] -> w509
                tunnel: [w594] -> w508
                i -> [w604]
                stop <- w605 stop-if-true
                n222 = Increment(x=w604) -> (x+1=w606:i32)
                n223 = call <vilib>:"WPI_MotorControlSetOutput.vi"("Output"=-1.0, "MotorControlDevRef"=w602) -> ("MotorControlDevRef"=w596:T5)  [unwired: 7 in, 2 out]
                n224 = Wait (ms)(milliseconds to wait=u32 25) -> ()  [unwired: 1 out]
                n225 = call <vilib>:"WPI_MotorControlSetOutput.vi"("Output"=1.0, "MotorControlDevRef"=w603) -> ("MotorControlDevRef"=w597:T5)  [unwired: 7 in, 2 out]
                n226 = Greater Or Equal?(x=w606, y=20) -> (x >= y?=w605:bool)
              }
              n227 = while {
                tunnel: w513 -> [w588]
                tunnel: w512 -> [w587]
                tunnel: [w584] -> _
                tunnel: w511 -> [w584]
                tunnel: w510 -> [w583]
                tunnel: [w583] -> w495
                tunnel: w509 -> [w582]
                tunnel: [w582] -> _
                tunnel: w508 -> [w581]
                tunnel: [w581] -> _
                i -> [w589]
                stop <- w590 stop-if-true
                n228 = Increment(x=w589) -> (x+1=w592:i32)
                n229 = call <vilib>:"WPI_MotorControlSetOutput.vi"("Output"=0.25, "MotorControlDevRef"=w587) -> ()  [unwired: 7 in, 3 out]
                n230 = call <vilib>:"WPI_MotorControlSetOutput.vi"("Output"=-0.25, "MotorControlDevRef"=w588) -> ()  [unwired: 7 in, 3 out]
                n231 = Wait (ms)(milliseconds to wait=u32 30) -> ()  [unwired: 1 out]
                n232 = Greater Or Equal?(x=w592, y=20) -> (x >= y?=w590:bool)
              }
              n233 = while {
                tunnel: w495 -> [w579]
                i -> [w574]
                stop <- w575 stop-if-true
                n234 = Increment(x=w574) -> (x+1=w576:i32)
                n235 = call-poly <vilib>:"WPI_RobotDriveArcadeDrive.vi"("Y axis value"=-0.75, "RobotDriveDevRef"=w579) -> ()  [unwired: 7 in, 3 out]
                n236 = Wait (ms)(milliseconds to wait=u32 20) -> ()  [unwired: 1 out]
                n237 = Greater Or Equal?(x=w576, y=20) -> (x >= y?=w575:bool)
              }
            }
          }
        }
        frame 1, Default {
          n238 = while {
            tunnel: w759 -> [w819]
            tunnel: [w817] -> _
            tunnel: [w816] -> w745
            tunnel: w758 -> [w816]
            tunnel: w757 -> [w815]
            tunnel: [w815] -> w742
            tunnel: w756 -> [w810]
            tunnel: w755 -> [w809]
            tunnel: [w809] -> _
            tunnel: [w810] -> _
            tunnel: [w812] -> w747
            tunnel: w748 -> [w812]
            i -> [w823]
            stop <- w820 stop-if-true
            n239 = Increment(x=w823) -> (x+1=w822:i32)
            n240 = Greater Or Equal?(x=w822, y=20) -> (x >= y?=w820:bool)
            n241 = Wait (ms)(milliseconds to wait=u32 75) -> ()  [unwired: 1 out]
            n242 = call-poly <vilib>:"WPI_RobotDriveArcadeDrive.vi"("Y axis value"=-0.75, "X axis value"=0.0, "RobotDriveDevRef"=w819) -> ("RobotDriveDevRef"=w817:T17)  [unwired: 6 in, 2 out]
            n243 = call <vilib>:"WPI_MotorControlSetOutput.vi"("Output"=-1.0, "MotorControlDevRef"=w809) -> ()  [unwired: 7 in, 3 out]
            n244 = call-poly <vilib>:"WPI_SolenoidSet.vi"("Value"=WPI_SolenoidValue."Forward", "SolenoidDevRef"=w810) -> ()  [unwired: 8 in, 2 out]
          }
          n245 = while {
            tunnel: w747 -> [w767]
            tunnel: [w767] -> w746
            tunnel: w745 -> [w766]
            tunnel: [w766] -> w744
            tunnel: [w765] -> w743
            tunnel: w742 -> [w765]
            i -> [w762]
            stop <- w761 stop-if-true
            n246 = Increment(x=w762) -> (x+1=w763:i32)
            n247 = Wait (ms)(milliseconds to wait=u32 25) -> ()  [unwired: 1 out]
            n248 = Greater Or Equal?(x=w763, y=20) -> (x >= y?=w761:bool)
          }
          n249 = while {
            tunnel: w744 -> [w802]
            tunnel: w743 -> [w803]
            tunnel: [w803] -> w754
            tunnel: [w802] -> w753
            tunnel: w746 -> [w800]
            i -> [w805]
            stop <- w804 stop-if-true
            n250 = call-poly <vilib>:"WPI_SolenoidGet.vi"("SolenoidDevRef"=w800) -> ("SolenoidDevRef"=w798:T12)  [unwired: 8 in, 2 out]
            n251 = Increment(x=w805) -> (x+1=w806:i32)
            n252 = Wait (ms)(milliseconds to wait=u32 50) -> ()  [unwired: 1 out]
            n253 = Greater Or Equal?(x=w806, y=20) -> (x >= y?=w804:bool)
            n254 = call-poly <vilib>:"WPI_SolenoidSet.vi"("Value"=WPI_SolenoidValue."Reverse", "SolenoidDevRef"=w798) -> ()  [unwired: 8 in, 2 out]
          }
          n255 = while {
            tunnel: w754 -> [w793]
            tunnel: w753 -> [w792]
            tunnel: [w791] -> w752
            tunnel: [w790] -> w751
            i -> [w795]
            stop <- w794 stop-if-true
            n256 = Increment(x=w795) -> (x+1=w797:i32)
            n257 = call <vilib>:"SD Read Number.vi"("Name"="AUTON-Shot") -> ("Numeric"=w786:dbl)  [unwired: 8 in, 2 out]
            n258 = Greater Or Equal?(x=w797, y=20) -> (x >= y?=w794:bool)
            n259 = Wait (ms)(milliseconds to wait=u32 50) -> ()  [unwired: 1 out]
            n260 = Divide(x=w786, y=100.0) -> (x/y=w785:dbl)
            n261 = Negate(x=w785) -> (-x=w787:dbl)
            n262 = call <vilib>:"WPI_MotorControlSetOutput.vi"("Output"=w787, "MotorControlDevRef"=w793) -> ("MotorControlDevRef"=w790:T5)  [unwired: 7 in, 2 out]
            n263 = call <vilib>:"WPI_MotorControlSetOutput.vi"("Output"=w785, "MotorControlDevRef"=w792) -> ("MotorControlDevRef"=w791:T5)  [unwired: 7 in, 2 out]
          }
          n264 = while {
            tunnel: w752 -> [w779]
            tunnel: w751 -> [w778]
            tunnel: [w779] -> w749
            tunnel: [w778] -> w750
            i -> [w780]
            stop <- w781 stop-if-true
            n265 = Increment(x=w780) -> (x+1=w782:i32)
            n266 = Wait (ms)(milliseconds to wait=u32 10) -> ()  [unwired: 1 out]
            n267 = Greater Or Equal?(x=w782, y=20) -> (x >= y?=w781:bool)
          }
          n268 = while {
            tunnel: w750 -> [w775]
            tunnel: w749 -> [w776]
            i -> [w770]
            stop <- w769 stop-if-true
            n269 = Increment(x=w770) -> (x+1=w772:i32)
            n270 = call <vilib>:"WPI_MotorControlSetOutput.vi"("Output"=0.1, "MotorControlDevRef"=w775) -> ()  [unwired: 7 in, 3 out]
            n271 = call <vilib>:"WPI_MotorControlSetOutput.vi"("Output"=-0.1, "MotorControlDevRef"=w776) -> ()  [unwired: 7 in, 3 out]
            n272 = Wait (ms)(milliseconds to wait=u32 100) -> ()  [unwired: 1 out]
            n273 = Greater Or Equal?(x=w772, y=20) -> (x >= y?=w769:bool)
          }
        }
      }
    }
    frame Disabled {
    }
  }
